vi "SubVI.vi"(8 "Grubość szyby":dbl=8.0, 9 "Szerokość":dbl=50.0, 10 "Długość":dbl=50.0, 11 "Wysokość":dbl=100.0) -> (0 "pH wody w ciągu 23 dni":dbl[](array[numeric]) format="%.2f", 1 "Wymagana ilość wody":dbl format="%.2g", 2 "Objętość netto":dbl format="%.2g", 3 "Objętość brutto":dbl format="%.2g", 4 "Rodzaje odczynów w\n       ciągu 23 dni":string[](array[string]))   [LabVIEW 2018]
doc: "Program zwraca informacje dotyczące akwarium i znajdującej się w nim wody. Po otrzymaniu od użytkownika danych: wysokość, długość, szerokość (wszystkie podawane w centymetrach) oraz grubości szkła (podawana w milimetrach) program liczy objętość brutto (teoretyczna, wyznaczona wyłącznie na podstawie wymiarów akwarium bez uwzględnienia grubości szkła), objętość netto (właściwa, wyznaczona z uwzglednieniem grubości szkła, które zawęża wewnętrzne wymiary) oraz wymagana ilość wody (minimalna wartość, będąca 90% objętości netto) - wszystkie te wartości wyrażone są w litrach. Dodatkowo program przeprowadza 23-dniową symulację współczynnika pH zmieniającego się dziennie o ±0,1-0,3 i przyjmując, że woda w momencie nalania do akwarium była idealne (pH=7) i odrazu w pierwszym dniu (po dodaniu np. ryb) zmieniła się. Wynikiem symulacji jest również tablica mówiąca czy dany współczynnik jest kwasowy, obojętny lub zasadowy."
panel:
  # "Wprowadź dane \ndotyczące akwarium"
  # "Informacje zwrotne"
  # "l"
  # "cm"
  # "l"
  # "cm"
  # "l"
  # "cm"
  # "mm"
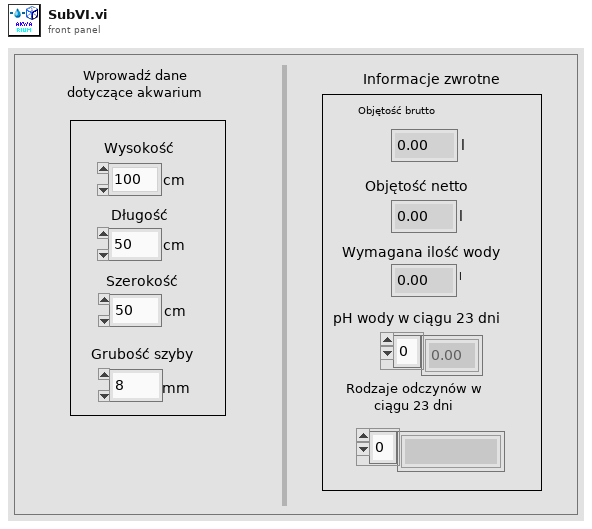
[diagram p1: front panel]
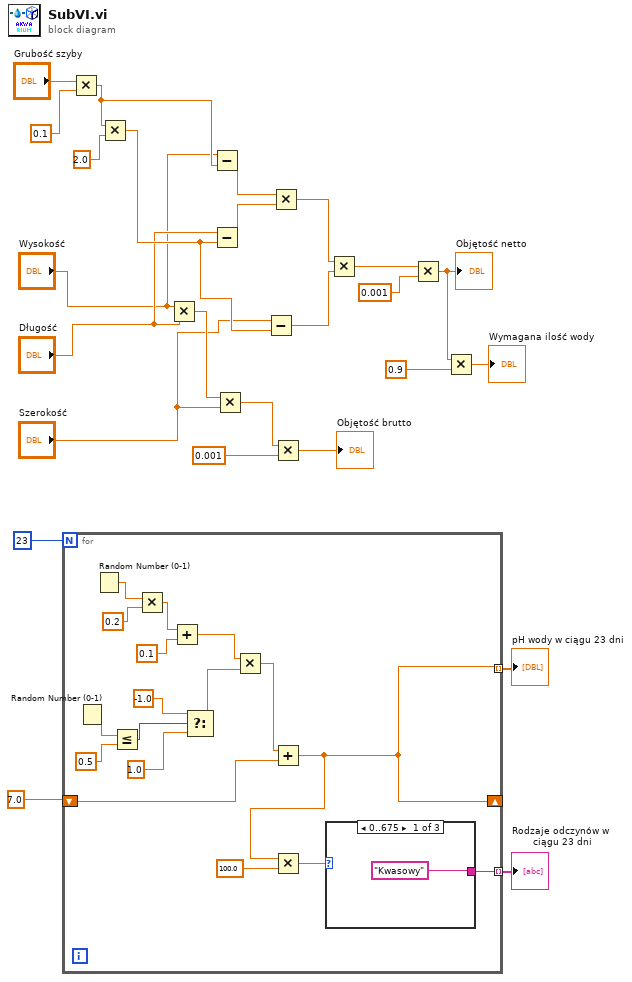
[diagram p0: block diagram]
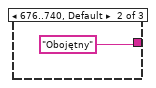
[diagram p2: hidden frame]
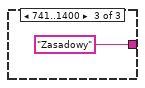
[diagram p3: hidden frame]
diagram:
  n1 = for {
    N: 23 -> [_]
    tunnel: [w28] -> w21 mode=indexing
    shift-right: [w28] -> _
    shift-left: 7.0 -> [w31]
    tunnel: [w29] -> w7 mode=indexing
    n2 = Random Number (0-1)() -> (number: 0 to 1=w37:dbl)
    n3 = Random Number (0-1)() -> (number: 0 to 1=w42:dbl)
    n4 = Less Or Equal?(x=w37, y=0.5) -> (x <= y?=w38:bool)
    n5 = Multiply(x=w42, y=0.2) -> (x*y=w40:dbl)
    n6 = Add(x=w40, y=0.1) -> (x+y=w33:dbl)
    n7 = Select(t=-1.0, s=w38, f=1.0) -> (s? t:f=w32:dbl)
    n8 = Multiply(x=w33, y=w32) -> (x*y=w30:dbl)
    n9 = Add(x=w30, y=w31) -> (x+y=w28:dbl)
    n10 = Multiply(x=w28, y=100.0) -> (x*y=w26:dbl)
    n11 = case shown="0..675" w26 {
      tunnel: ["Kwasowy" "Obojętny" "Zasadowy"] -> w29
      frame 0..675 {
      }
      frame 676..740, Default {
      }
      frame 741..1400 {
      }
    }
  }
  "pH wody w ciągu 23 dni" <- w21
  "Rodzaje odczynów w\n       ciągu 23 dni" <- w7
  n12 = Multiply(x="Grubość szyby", y=0.1) -> (x*y=w4:dbl)
  n13 = Multiply(x=w4, y=2.0) -> (x*y=w5:dbl)
  n14 = Multiply(x="Wysokość", y="Długość") -> (x*y=w25:dbl)
  n15 = Subtract(x="Wysokość", y=w4) -> (x-y=w18:dbl)
  n16 = Subtract(x="Długość", y=w5) -> (x-y=w17:dbl)
  n17 = Multiply(x=w25, y="Szerokość") -> (x*y=w24:dbl)
  n18 = Subtract(x="Szerokość", y=w5) -> (x-y=w16:dbl)
  n19 = Multiply(x=w18, y=w17) -> (x*y=w15:dbl)
  n20 = Multiply(x=w24, y=0.001) -> (x*y=→"Objętość brutto":dbl)
  n21 = Multiply(x=w15, y=w16) -> (x*y=w14:dbl)
  n22 = Multiply(x=w14, y=0.001) -> (x*y=w8:dbl)
  "Objętość netto" <- w8
  n23 = Multiply(x=w8, y=0.9) -> (x*y=→"Wymagana ilość wody":dbl)
